vi "Test_oven_T.vi"() -> ()   [LabVIEW 2016]
panel:
  out "Omega T error":errorcluster
  in  "stop":bool
  out "Omega Iteration":i32
  in  "byte count":u32=15
  out "Oven Temp":dbl
  out "Oven Temperature":dbl(graph)
  out "Omega read buffer":string
  in  "Wait (ms)":u32=500
  in  "Omega VISA resource":refnum<visa-resource-name>="TCPIP0::192.168.1.160::966::SOCKET"
  out "Read errors":i32
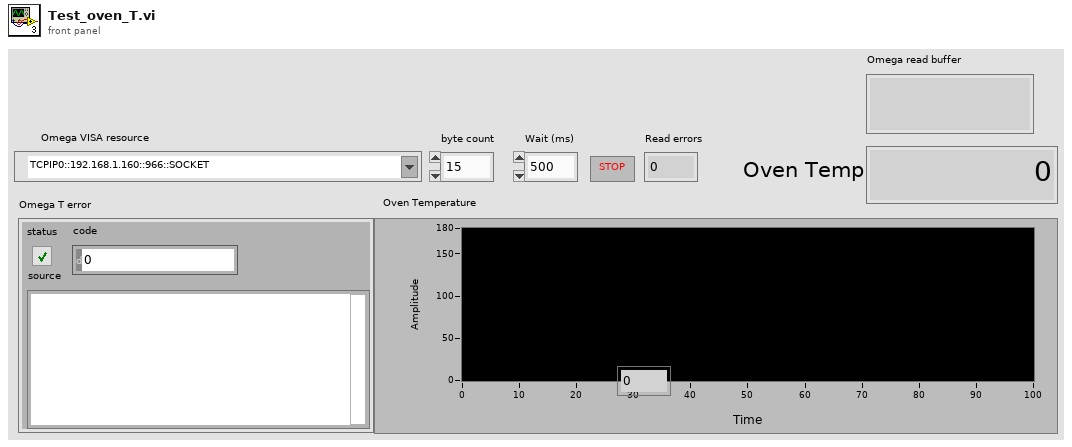
[diagram p1: front panel]
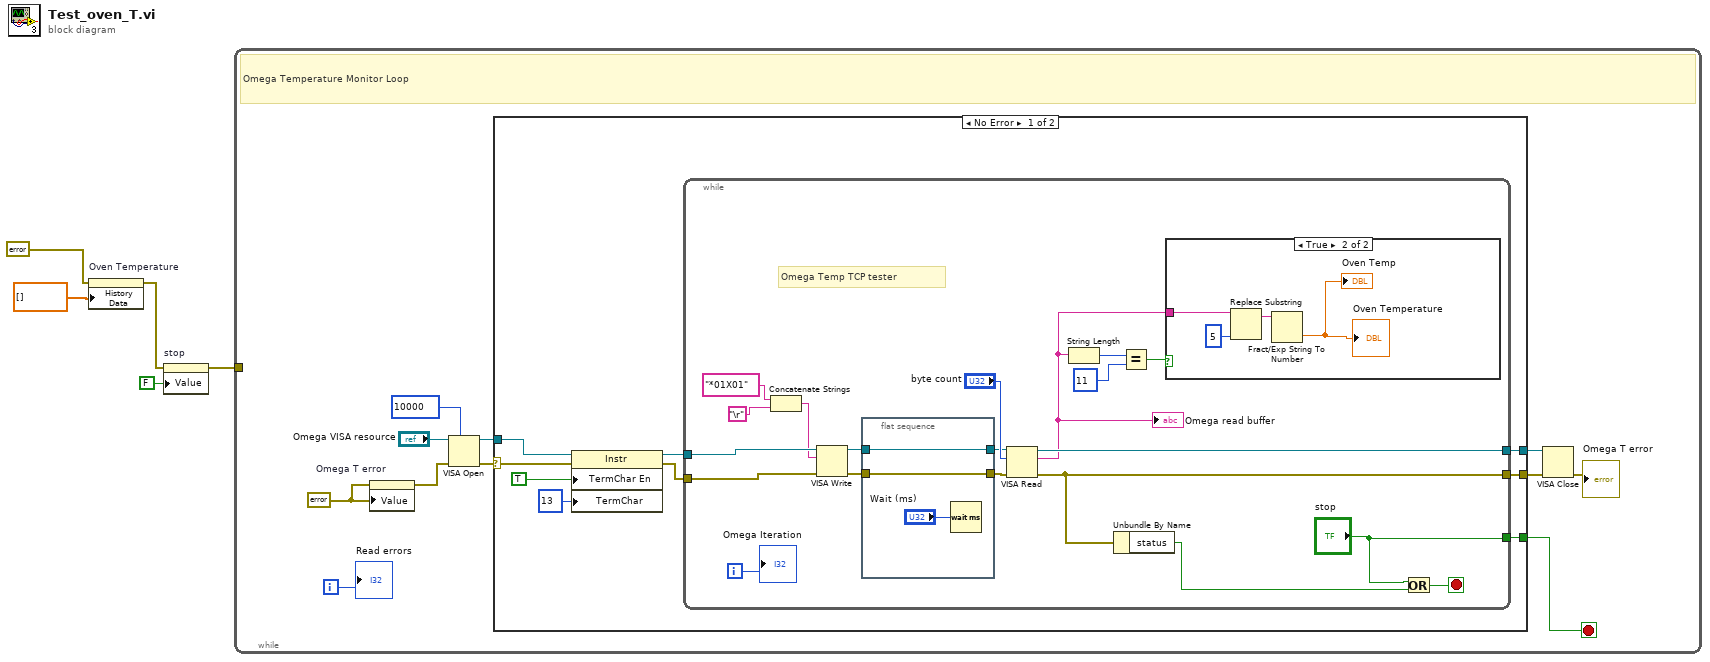
[diagram p0: block diagram]
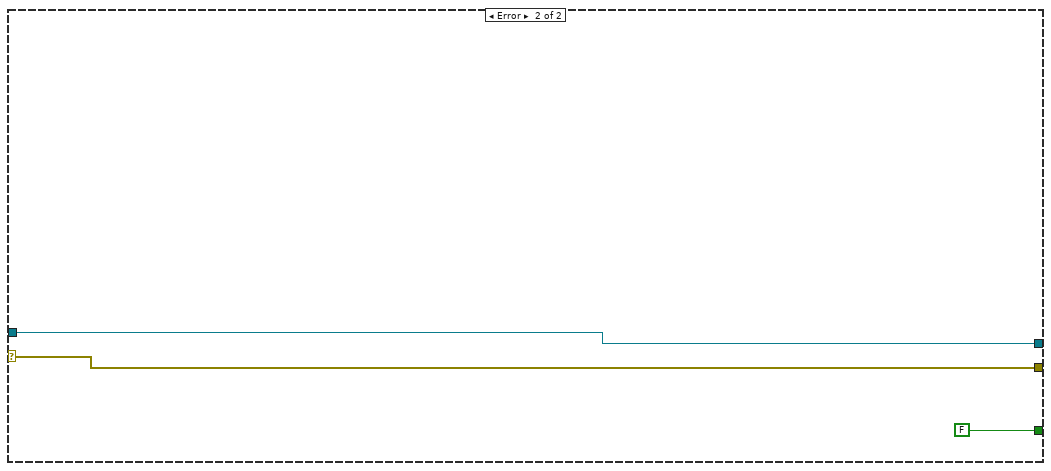
[diagram p3: hidden frame]
diagram:
  n1 = property on="Oven Temperature" class="WFChart (strict)"(error in=errorcluster {"status"=FALSE, "code"=0, "source"=""} ("error in (no error)"), "History Data"=dbl[] []) -> (error out=w3:errorcluster)  [unwired: 1 in, 1 out]
  n2 = property on="stop" class="Bool (strict)"(error in=w3, "Value"=FALSE ("stop")) -> (error out=w1:errorcluster)  [unwired: 1 in, 1 out]
  n3 = while {
    tunnel: w1 -> [_]
    i -> [w7]
    stop <- w8 stop-if-true
    w10 = errorcluster {"status"=FALSE, "code"=0, "source"=""} ("error in (no error)")
    # "Omega Temperature Monitor Loop"
    n4 = property on="Omega T error" class="Clust (strict)"(error in=w10, "Value"=w10) -> (error out=w12:errorcluster)  [unwired: 1 in, 1 out]
    n5 = VISA Open(timeout (0)=u32 10000 ("VISA Open timeout (0)"), error in (no error)=w12, VISA resource name="Omega VISA resource") -> (VISA resource name=w16:refnum<visa-resource-name>, error out=w6:errorcluster)  [unwired: 2 in]
    n6 = case shown="No Error" w6 {
      selector: w6 -> [w18 w53]
      tunnel: w16 -> [w23 w55]
      tunnel: [w25 w55] -> w15
      tunnel: [w24 w53] -> w14
      tunnel: [w19 FALSE ("stop")] -> w8
      frame No Error {
        n7 = property class="Instr"(reference=w23, error in=w18, "TermChar En"=TRUE ("Message Based Settings:Termination Character Enable"), "TermChar"=u8 13 ("Message Based Settings:Termination Character")) -> (reference out=w22:refnum<visa-resource-name>, error out=w17:errorcluster)
        n8 = while {
          tunnel: w22 -> [w41]
          tunnel: [w45] -> w25
          tunnel: w17 -> [w36]
          tunnel: [w44] -> w24
          tunnel: ["stop"] -> w19
          i -> [w42]
          stop <- w43 stop-if-true
          # "Omega Temp TCP tester"
          n9 = Concatenate Strings("*01X01" ("data in"), "\r") -> (w38:string)
          n10 = VISA Write(VISA resource name=w41, write buffer=w38, error in (no error)=w36) -> (VISA resource name out=w29:refnum<visa-resource-name>, error out=w31:errorcluster)  [unwired: 1 out]
          n11 = flat-sequence {
            tunnel: w31 -> [w48]
            tunnel: [w48] -> w30
            tunnel: w29 -> [w47]
            tunnel: [w47] -> w28
            frame #0 {
              n12 = Wait (ms)(milliseconds to wait="Wait (ms)") -> ()  [unwired: 1 out]
            }
          }
          n13 = VISA Read(VISA resource name=w28, byte count="byte count", error in (no error)=w30) -> (VISA resource name out=w45:refnum<visa-resource-name>, read buffer=w32:string, error out=w44:errorcluster)  [unwired: 1 out]
          "Omega read buffer" <- w32
          n14 = String Length(string=w32) -> (length=w35:i32)
          n15 = Unbundle By Name(w44) -> ("status"=w27:bool)
          n16 = Equal?(x=w35, y=11) -> (x = y?=w33:bool)
          n17 = case shown="True" w33 {
            tunnel: w32 -> [_ w49]
            frame False {
            }
            frame True {
              n18 = Replace Substring(2:5 ("length (len. of substring)"), 5:w49) -> (1:w50:string)  [unwired: 2 in, 1 out]
              n19 = Fract/Exp String To Number(string=w50) -> (number=→"Oven Temp" →"Oven Temperature":dbl)  [unwired: 3 in, 1 out]
            }
          }
          n20 = Or(x="stop", y=w27) -> (x .or. y?=w43:bool)
          "Omega Iteration" <- w42
        }
      }
      frame Error {
      }
    }
    n21 = VISA Close(VISA resource name=w15, error in (no error)=w14) -> (error out=→"Omega T error":errorcluster)
    "Read errors" <- w7
  }
